vi "seconds_to_time.vi"(10 "# Seconds (0)":u32) -> (2 "Elapsed Time (00:00:00)":string="00:00:00")   [LabVIEW 2012]
doc: "This VI takes an integer input of a number of seconds. It converts this to a string output of the amount of time represented in days, hours, minutes and seconds.\n\nOutput is in format\n [DD] HH:MM:SS ([days] hours:minutes:seconds)\n\nThe number of days appears only if the period # of seconds is greater than or equal to 86400, or 24 hours.\n\nThis VI was created in LabVIEW 6.1"
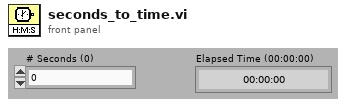
[diagram p1: front panel]
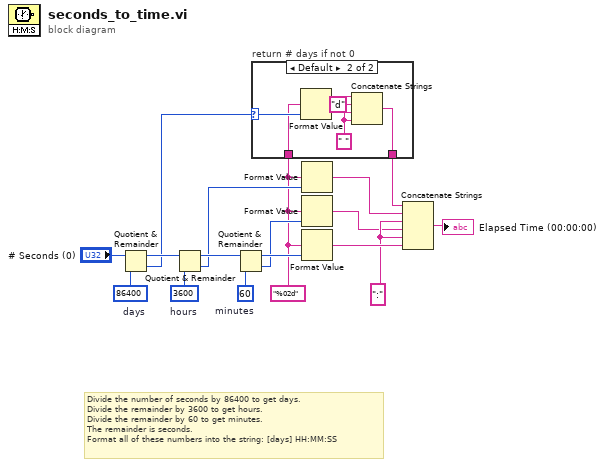
[diagram p0: block diagram]
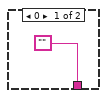
[diagram p2: hidden frame]
diagram:
  w4 = u32 86400  # days
  w1 = "%02d" ("format string")
  w13 = ":"
  w16 = u32 3600  # hours
  w15 = u32 60  # minutes
  # "Divide the number of seconds by 86400 to get days.\nDivide the remainder by 3600 to get hours.\nDivide the remainder by 60 to get minutes.\nThe remainder is seconds.\nFormat all of these numbers into the string: [days] HH:MM:SS"
  n1 = Quotient & Remainder(x="# Seconds (0)", y=w4) -> (x-y*floor(x/y)=w6:u32, floor(x/y)=w3:u32)
  n2 = Quotient & Remainder(x=w6, y=w16) -> (x-y*floor(x/y)=w17:u32, floor(x/y)=w8:u32)
  n3 = Quotient & Remainder(x=w17, y=w15) -> (x-y*floor(x/y)=w9:u32, floor(x/y)=w7:u32)
  n4 = case "return # days if not 0" shown="Default" w3 {
    selector: w3 -> [_ w24]
    tunnel: ["" w22] -> w2
    tunnel: w1 -> [_ w21]
    frame 0 {
    }
    frame Default {
      w23 = " "
      n5 = Format Value(format string=w21, value (0)=w24) -> (output string=w20:string)  [unwired: 1 in]
      n6 = Concatenate Strings(w20, "d" ("string"), w23, w23) -> (w22:string)
    }
  }
  n7 = Format Value(format string=w1, value (0)=w8) -> (output string=w10:string)  [unwired: 1 in]
  n8 = Format Value(format string=w1, value (0)=w7) -> (output string=w11:string)  [unwired: 1 in]
  n9 = Format Value(format string=w1, value (0)=w9) -> (output string=w14:string)  [unwired: 1 in]
  n10 = Concatenate Strings(w2, w10, w13, w11, w13, w14) -> (→"Elapsed Time (00:00:00)":string)
